vi "Update Menu Items.vi"(8 "error in (no error)":errorcluster, 9 "Coords":T1, 10 "MenuRef":refnum<k9>, 11 "Table in":refnum<vi>) -> (0 "error out":errorcluster)   [LabVIEW 2014, in "SLSC configuration System Explorer.lvlib"]
uses:
  SLSC configuration System Explorer.lvlib
  <vilib>/Utility/miscctls.llb/LVPoint32TypeDef.ctl
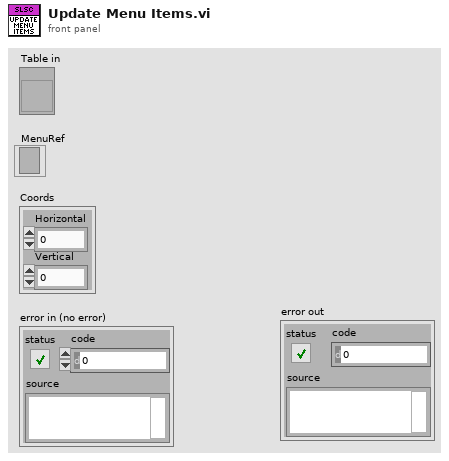
[diagram p1: front panel]
types:
  T1 = typedef "LVPoint32TypeDef.ctl" = cluster{"Horizontal":i32, "Vertical":i32}
  T2 = typedef "LVRowAndColumnTypeDef.ctl" = cluster{"Row":i32, "Column":i32}
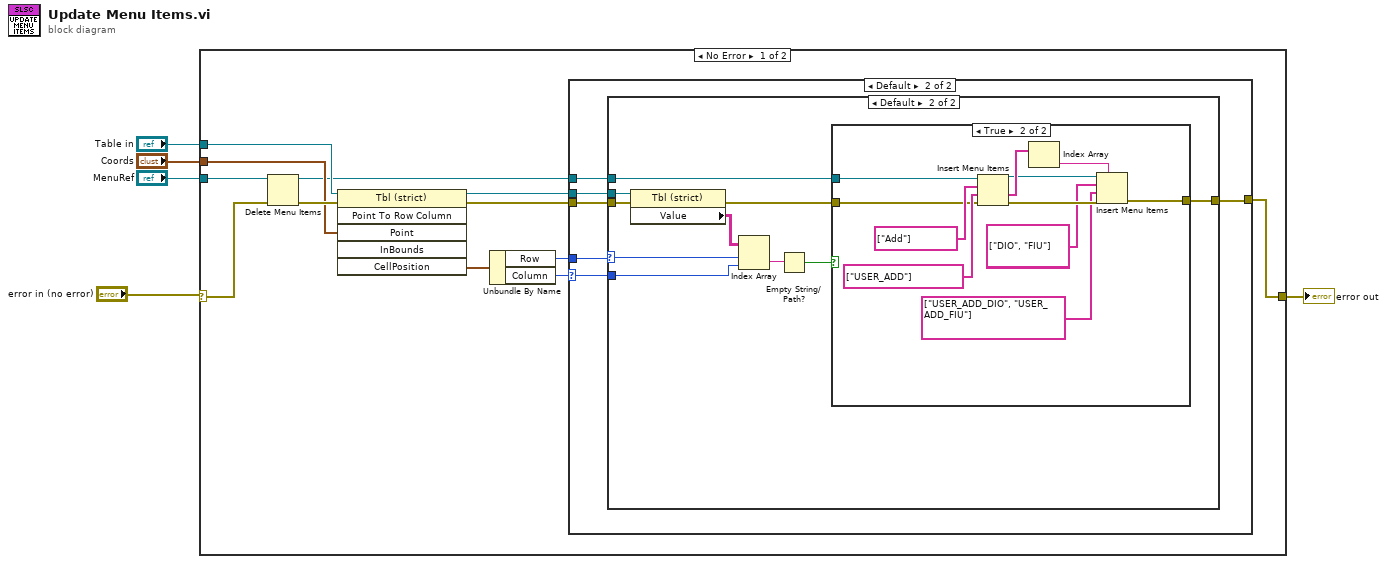
[diagram p0: block diagram]
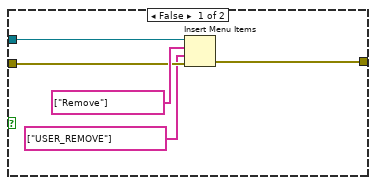
[diagram p4: hidden frame]
diagram:
  n1 = case shown="No Error" "error in (no error)" {
    selector: "error in (no error)" -> [w6 w52]
    tunnel: "MenuRef" -> [w16 _]
    tunnel: "Coords" -> [w15 _]
    tunnel: "Table in" -> [w14 _]
    tunnel: [w7 w52] -> w2
    frame No Error {
      n2 = Delete Menu Items(6:w6, 9:w16) -> (0:w17:errorcluster, 3:w10:refnum<k9>)  [unwired: 2 in]
      n3 = invoke class="Tbl (strict)" method="Point To Row Column"(reference=w14, error in=w17, "Point"=w15) -> (reference out=w8:refnum<vi>, error out=w9:errorcluster, "CellPosition"=w13:T2)  [unwired: 3 in, 3 out]
      n4 = Unbundle By Name(w13) -> ("Row"=w11:i32, "Column"=w12:i32)
      n5 = case shown="Default" w12 {
        selector: w12 -> [_ w20]
        tunnel: w11 -> [_ w24]
        tunnel: w10 -> [_ w23]
        tunnel: w9 -> [w18 w22]
        tunnel: w8 -> [_ w21]
        tunnel: [w18 w19] -> w7
        frame 0, 1 {
          # "No menu items for columns 0 and 1"
        }
        frame Default {
          n6 = case shown="Default" w24 {
            selector: w24 -> [_ w31]
            tunnel: w23 -> [_ w35]
            tunnel: w22 -> [w25 w34]
            tunnel: w21 -> [_ w33]
            tunnel: w20 -> [_ w30]
            tunnel: [w25 w26] -> w19
            frame 0 {
              # "No menu items for row 0"
            }
            frame Default {
              n7 = property class="Tbl (strict)"(reference=w33, error in=w34) -> (error out=w27:errorcluster, "Value"=w32:string[][])  [unwired: 1 out]
              n8 = Index Array(array=w32, index (row)=w31, index (col)=w30) -> (element=w29:string)
              n9 = Empty String/Path?(string/path=w29) -> (empty?=w28:bool)
              n10 = case shown="True" w28 {
                tunnel: w35 -> [w38 w51]
                tunnel: w27 -> [w39 w41]
                tunnel: [w36 w44] -> w26
                frame False {
                  n11 = Insert Menu Items(6:w39, 7:string[] ["USER_REMOVE"] ("item names"), 8:string[] ["Remove"] ("item names"), 9:w38) -> (0:w36:errorcluster)  [unwired: 2 in, 2 out]
                }
                frame True {
                  (unwired) string[] ["DIO", "FIU"] ("item names")
                  n12 = Insert Menu Items(6:w41, 7:string[] ["USER_ADD"] ("item tags"), 8:string[] ["Add"] ("item names"), 9:w51) -> (0:w49:errorcluster, 1:w50:string[], 3:w48:refnum<k9>)  [unwired: 2 in]
                  n13 = Index Array(array=w50) -> (element=w47:string)  [unwired: 1 in]
                  n14 = Insert Menu Items(5:w47, 6:w49, 7:string[] ["USER_ADD_DIO", "USER_ADD_FIU"] ("item tags"), 8:string[] ["DIO", "FIU"] ("item names"), 9:w48) -> (0:w44:errorcluster)  [unwired: 1 in, 2 out]
                }
              }
            }
          }
        }
      }
    }
    frame Error {
    }
  }
  "error out" <- w2
